vi "Refresh List Length.vi"(8 "error in (no error)":errorcluster caption="Error In", 9 "H":bool, 11 "V":bool) -> (0 "error out":errorcluster caption="Error Out", 3 "Array":u32[](array[numeric]))   [LabVIEW 2020]
panel:
  out "Left":u32[](array[numeric])
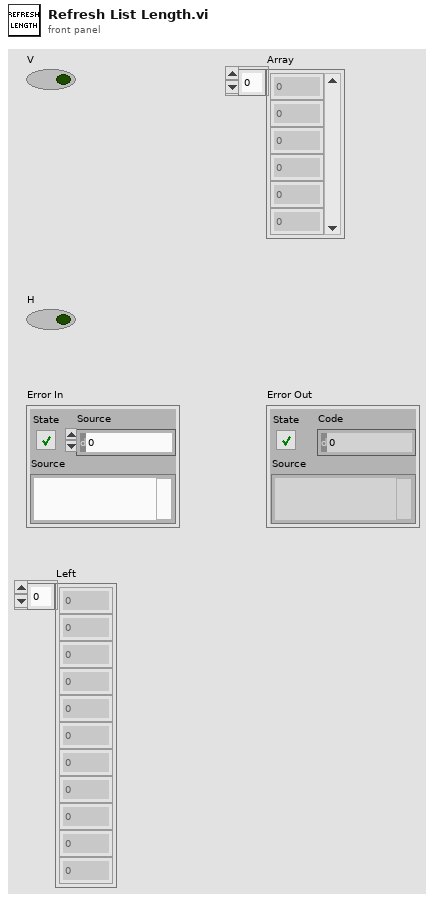
[diagram p1: front panel]
types:
  T1 = enum8{"Enabled", "Disabled", "Disabled and Grayed Out"}
  T2 = enum16{"Always On", "Always Off", "Off While Running"}
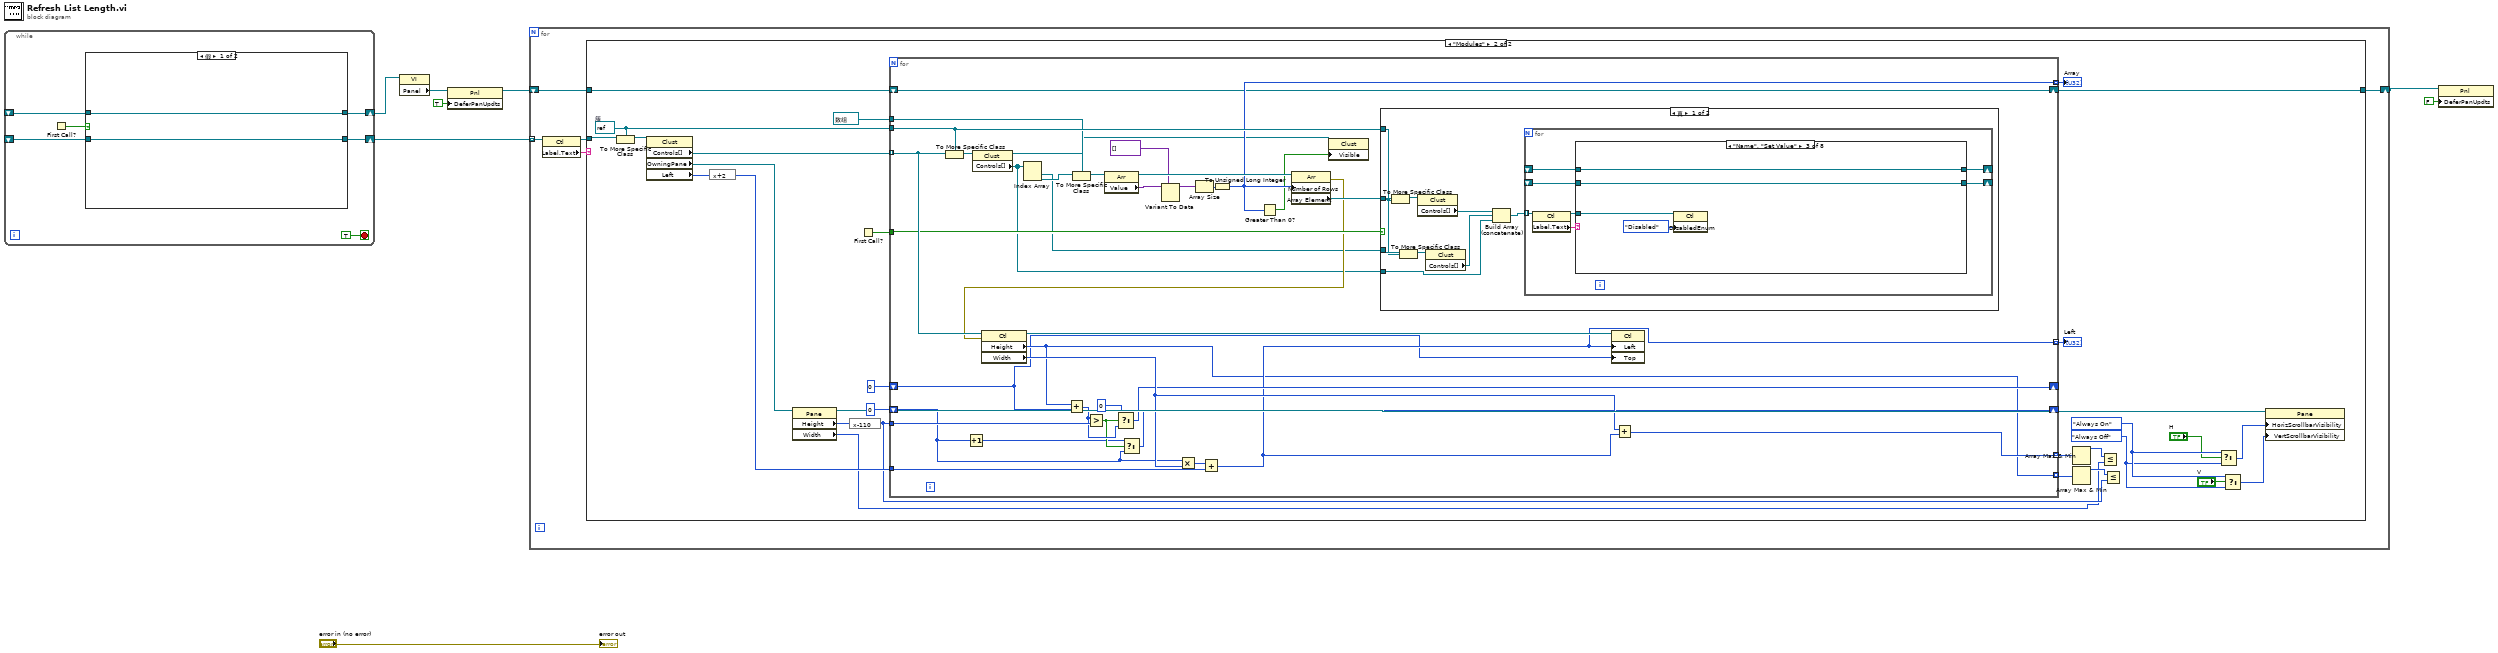
[diagram p0: block diagram]
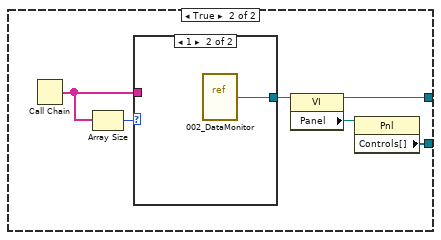
[diagram p2: hidden frame]
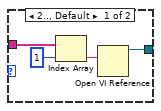
[diagram p3: hidden frame]
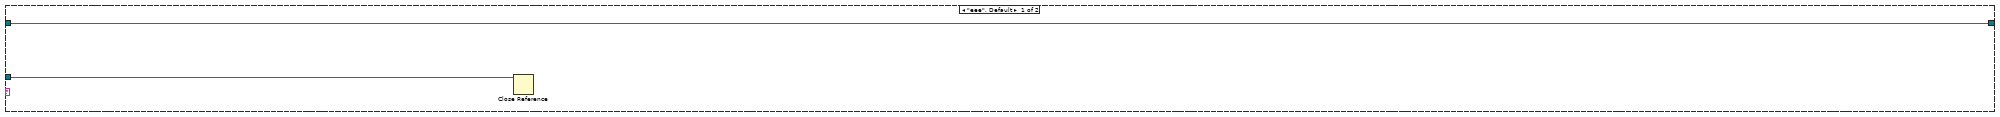
[diagram p4: hidden frame]
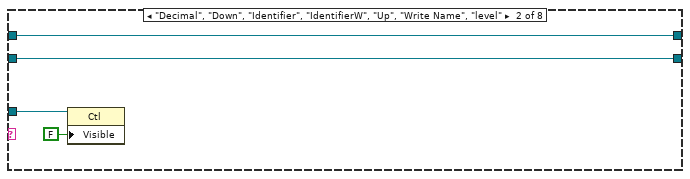
[diagram p6: hidden frame]
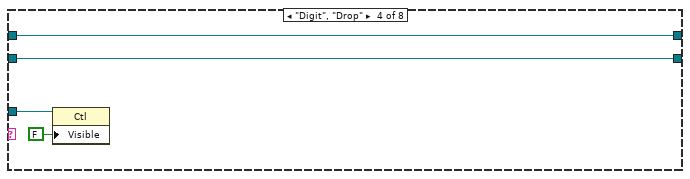
[diagram p7: hidden frame]
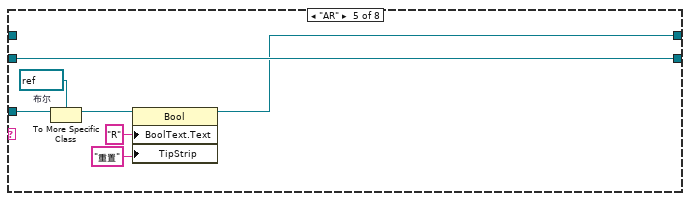
[diagram p8: hidden frame]
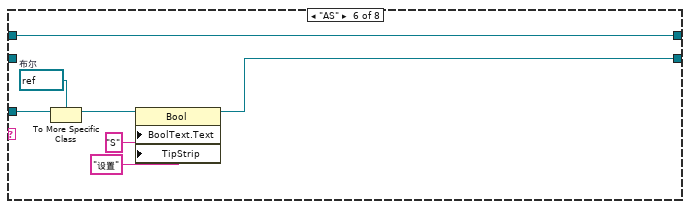
[diagram p9: hidden frame]
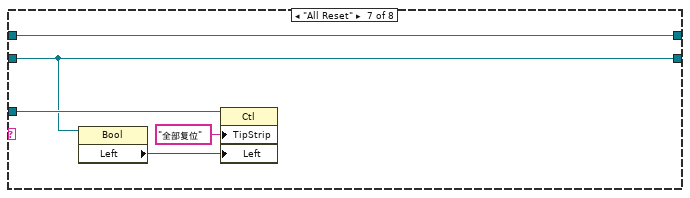
[diagram p10: hidden frame]
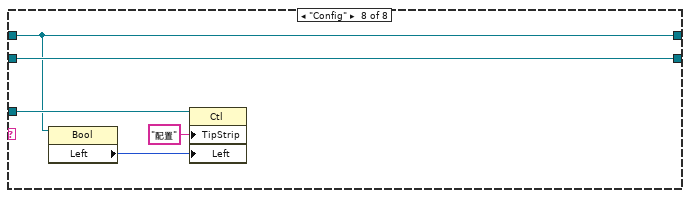
[diagram p11: hidden frame]
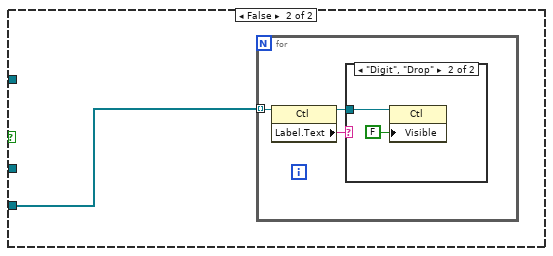
[diagram p12: hidden frame]
diagram:
  n1 = while {
    shift-right: [w14] -> w7
    shift-left: _ -> [w11]
    shift-right: [w10] -> w6
    shift-left: _ -> [w9]
    stop <- TRUE stop-if-true
    n2 = First Call?() -> (First Call?: T/F=w13:bool)
    n3 = case shown="假" w13 {
      tunnel: [w16 w22] -> w14
      tunnel: w11 -> [w16 _]
      tunnel: [w15 w17] -> w10
      tunnel: w9 -> [w15 _]
      frame False {
      }
      frame True {
        n4 = Call Chain() -> (call chain=w20:string[])
        n5 = Array Size(array=w20) -> (size(s)=w21:i32)
        n6 = case shown="1" w21 {
          tunnel: [w24 w27] -> w18
          tunnel: w20 -> [w23 _]
          frame 2.., Default {
            n7 = Index Array(array=w23, index=1 ("索引")) -> (element=w25:string)
            n8 = Open VI Reference(vi path=w25) -> (vi reference=w24:refnum<vi>)  [unwired: 5 in, 1 out]
          }
          frame 1 {
            n9 = vi-ref "002_DataMonitor.vi"() -> (w27:refnum<vi>)
          }
        }
        n10 = property class="VI"(reference=w18) -> (reference out=w17:refnum<vi>, "Panel"=w19:refnum<vi>)  [unwired: 1 in, 1 out]
        n11 = property class="Pnl"(reference=w19) -> ("Controls[]"=w22:refnum<vi>[])  [unwired: 1 in, 2 out]
      }
    }
  }
  n12 = property class="VI"(reference=w6) -> ("Panel"=w5:refnum<vi>)  [unwired: 1 in, 2 out]
  n13 = property class="Pnl"(reference=w5, "DeferPanUpdts"=TRUE ("延迟前面板更新")) -> (reference out=w3:refnum<vi>)  [unwired: 1 in, 1 out]
  n14 = for {
    tunnel: w7 -> [w32] mode=indexing
    shift-right: [w28] -> w1
    shift-left: w3 -> [w29]
    n15 = property class="Ctl"(reference=w32) -> (reference out=w30:refnum<vi>, "Label.Text"=w31:string)  [unwired: 1 in, 1 out]
    n16 = case shown="\"Modules\"" w31 {
      tunnel: w30 -> [w34 w63]
      tunnel: w29 -> [w33 w40]
      tunnel: [w33 w39] -> w28
      frame "eee", Default {
        n17 = Close Reference(reference=w34) -> ()  [unwired: 1 in, 1 out]
      }
      frame "Modules" {
        w41 = T2."Always Off" ("垂直滚动条可见")
        w42 = T2."Always On" ("垂直滚动条可见")
        w61 = refnum<vi> refnum  # 簇
        n18 = To More Specific Class(target class=w61, reference=w63) -> (specific class reference=w62:refnum<vi>)  [unwired: 1 in, 1 out]
        n19 = property on="属性节点" class="Clust"(reference=w62) -> ("Controls[]"=w58:refnum<vi>[], "OwningPane"=w59:refnum<vi>, "Left"=w57:i32)  [unwired: 1 in, 2 out]
        n20 = expression code="x+2"(w57) -> (w53:i32)
        n21 = property class="Pane"(reference=w59) -> (reference out=w51:refnum<vi>, "Height"=w56:u32, "Width"=w45:u32)  [unwired: 1 in, 1 out]
        n22 = expression code="x-110"(w56) -> (w46:u32)
        n23 = First Call?() -> (First Call?: T/F=w52:bool)
        n24 = for {
          tunnel: w58 -> [w95] mode=indexing
          tunnel: w61 -> [w99]
          tunnel: refnum<vi> refnum ("Data") -> [w98]
          tunnel: w46 -> [w97]
          tunnel: w53 -> [w96]
          shift-right: [w77] -> _
          shift-left: u32 0 -> [w66]
          shift-right: [w68] -> _
          shift-left: u32 0 -> [w76]
          tunnel: w52 -> [w82]
          tunnel: [w67] -> w49 mode=indexing
          tunnel: [w80] -> w50 mode=indexing
          tunnel: [w74] -> w44 mode=indexing
          tunnel: [w69] -> w43 mode=indexing
          shift-right: [w64] -> w39
          shift-left: w40 -> [w64]
          n25 = To More Specific Class(target class=w99, reference=w95) -> (specific class reference=w90:refnum<vi>)  [unwired: 1 in, 1 out]
          n26 = Increment(x=w76) -> (x+1=w65:u32)
          n27 = property on="属性节点" class="Clust"(reference=w90) -> (reference out=w73:refnum<vi>, "Controls[]"=w75:refnum<vi>[])  [unwired: 1 in, 1 out]
          n28 = Index Array(array=w75) -> (element #1=w70:refnum<vi>, element #2=w71:refnum<vi>)  [unwired: 2 in]
          n29 = To More Specific Class(target class=w98, reference=w71) -> (specific class reference=w89:refnum<vi>)  [unwired: 1 in, 1 out]
          n30 = property class="Arr"(reference=w89) -> (reference out=w88:refnum<vi>, "Value"=w85:variant)  [unwired: 1 in, 1 out]
          n31 = Variant To Data(type=variant[] [], Variant=w85) -> (data=w83:variant[])  [unwired: 1 in, 1 out]
          n32 = Array Size(array=w83) -> (size(s)=w87:i32)
          n33 = To Unsigned Long Integer(number=w87) -> (unsigned 32bit integer=w74:u32)
          n34 = Greater Than 0?(x=w74) -> (x > 0?=w72:bool)
          n35 = property class="Arr"(reference=w88, "Number of Rows"=w74) -> (error out=w81:errorcluster, "Array Element"=w86:refnum<vi>)  [unwired: 1 in, 1 out]
          n36 = property class="Ctl"(reference=w95, error in=w81) -> (reference out=w91:refnum<vi>, "Height"=w67:u32, "Width"=w78:u32)  [unwired: 1 out]
          n37 = Add(x=w67, y=w66) -> (x+y=w93:u32)
          n38 = Greater?(x=w93, y=w97) -> (0:w79:bool)
          n39 = Select(t=u32 0, s=w79, f=w93) -> (s? t:f=w77:u32)
          n40 = Select(t=w65, s=w79, f=w76) -> (s? t:f=w68:u32)
          n41 = Multiply(x=w76, y=w78) -> (x*y=w92:u32)
          n42 = Add(x=w92, y=w96) -> (x+y=w69:u32)
          n43 = property class="Clust"(reference=w73, "Visible"=w72) -> ()  [unwired: 1 in, 2 out]
          n44 = case shown="真" w82 {
            tunnel: w99 -> [w102 _]
            tunnel: w86 -> [w107 _]
            tunnel: w70 -> [w103 _]
            tunnel: w75 -> [w100 w154]
            frame True {
              n45 = To More Specific Class(target class=w102, reference=w107) -> (specific class reference=w108:refnum<vi>)  [unwired: 1 in, 1 out]
              n46 = To More Specific Class(target class=w102, reference=w103) -> (specific class reference=w104:refnum<vi>)  [unwired: 1 in, 1 out]
              n47 = property on="属性节点" class="Clust"(reference=w108) -> ("Controls[]"=w106:refnum<vi>[])  [unwired: 1 in, 2 out]
              n48 = property on="属性节点" class="Clust"(reference=w104) -> ("Controls[]"=w101:refnum<vi>[])  [unwired: 1 in, 2 out]
              n49 = Build Array (concatenate)(w106, w101, w100) -> (w105:refnum<vi>[])
              n50 = for {
                tunnel: w105 -> [w115] mode=indexing
                shift-right: [w112] -> _
                shift-left: _ -> [w111]
                shift-right: [w110] -> _
                shift-left: _ -> [w109]
                n51 = property class="Ctl"(reference=w115) -> (reference out=w113:refnum<vi>, "Label.Text"=w114:string)  [unwired: 1 in, 1 out]
                n52 = case shown="\"Name\", \"Set Value\"" w114 {
                  tunnel: w113 -> [_ w121 w123 w129 w136 w143 w148 w153]
                  tunnel: [w117 w119 w125 w127 w130 w138 w146 w150] -> w112
                  tunnel: w111 -> [w117 w119 w125 w127 _ w138 w146 w150]
                  tunnel: [w116 w118 w124 w126 w131 w137 w145 w151] -> w110
                  tunnel: w109 -> [w116 w118 w124 w126 w131 _ w145 w151]
                  frame "eee", Default {
                  }
                  frame "Decimal", "Down", "Identifier", "IdentifierW", "Up", "Write Name", "level" {
                    n53 = property class="Ctl"(reference=w121, "Visible"=FALSE ("可见")) -> ()  [unwired: 1 in, 2 out]
                  }
                  frame "Name", "Set Value" {
                    n54 = property class="Ctl"(reference=w123, "DisabledEnum"=T1."Disabled" ("禁用")) -> ()  [unwired: 1 in, 2 out]
                  }
                  frame "Digit", "Drop" {
                    n55 = property class="Ctl"(reference=w129, "Visible"=FALSE ("可见")) -> ()  [unwired: 1 in, 2 out]
                  }
                  frame "AR" {
                    w135 = refnum<vi> refnum  # 布尔
                    n56 = To More Specific Class(target class=w135, reference=w136) -> (specific class reference=w134:refnum<vi>)  [unwired: 1 in, 1 out]
                    n57 = property class="Bool"(reference=w134, "BoolText.Text"="R" ("布尔文本.文本"), "TipStrip"="重置" ("说明信息")) -> (reference out=w130:refnum<vi>)  [unwired: 1 in, 1 out]
                  }
                  frame "AS" {
                    w142 = refnum<vi> refnum  # 布尔
                    n58 = To More Specific Class(target class=w142, reference=w143) -> (specific class reference=w141:refnum<vi>)  [unwired: 1 in, 1 out]
                    n59 = property class="Bool"(reference=w141, "BoolText.Text"="S" ("布尔文本.文本"), "TipStrip"="设置" ("说明信息")) -> (reference out=w137:refnum<vi>)  [unwired: 1 in, 1 out]
                  }
                  frame "All Reset" {
                    n60 = property class="Bool"(reference=w145) -> ("Left"=w144:i32)  [unwired: 1 in, 2 out]
                    n61 = property class="Ctl"(reference=w148, "TipStrip"="全部复位" ("说明信息"), "Left"=w144) -> ()  [unwired: 1 in, 2 out]
                  }
                  frame "Config" {
                    n62 = property class="Bool"(reference=w150) -> ("Left"=w149:i32)  [unwired: 1 in, 2 out]
                    n63 = property class="Ctl"(reference=w153, "TipStrip"="配置" ("说明信息"), "Left"=w149) -> ()  [unwired: 1 in, 2 out]
                  }
                }
              }
            }
            frame False {
              n64 = for {
                tunnel: w154 -> [w157] mode=indexing
                n65 = property class="Ctl"(reference=w157) -> (reference out=w155:refnum<vi>, "Label.Text"=w156:string)  [unwired: 1 in, 1 out]
                n66 = case shown="\"Digit\", \"Drop\"" w156 {
                  tunnel: w155 -> [_ w159]
                  frame "eee", Default {
                  }
                  frame "Digit", "Drop" {
                    n67 = property class="Ctl"(reference=w159, "Visible"=FALSE ("可见")) -> ()  [unwired: 1 in, 2 out]
                  }
                }
              }
            }
          }
          n68 = property class="Ctl"(reference=w91, "Left"=w69, "Top"=w66) -> ()  [unwired: 1 in, 2 out]
          n69 = Add(x=w78, y=w69) -> (x+y=w80:u32)
        }
        "Array" <- w44
        "Left" <- w43
        n70 = Array Max & Min(array=w50) -> (max value=w48:u32)  [unwired: 3 out]
        n71 = Array Max & Min(array=w49) -> (max value=w47:u32)  [unwired: 3 out]
        n72 = Less Or Equal?(x=w48, y=w45) -> ()  [unwired: 1 out]
        n73 = Less Or Equal?(x=w47, y=w46) -> ()  [unwired: 1 out]
        n74 = Select(t=w42, s="H", f=w41) -> (s? t:f=w38:T2)
        n75 = Select(t=w42, s="V", f=w41) -> (s? t:f=w37:T2)
        n76 = property class="Pane"(reference=w51, "HorizScrollbarVisibility"=w38, "VertScrollbarVisibility"=w37) -> ()  [unwired: 1 in, 2 out]
      }
    }
  }
  n77 = property class="Pnl"(reference=w1, "DeferPanUpdts"=FALSE ("延迟前面板更新")) -> ()  [unwired: 1 in, 2 out]
  "error out" <- "error in (no error)"
